vi "Create.vi"(8 "error in (no error)":errorcluster, 10 "GPIO":refnum<class "GPIO.lvclass">, 11 "ADC #":T1=-1) -> (0 "error out":errorcluster, 3 "AnalogIn out":refnum<class "AI.lvclass">)   [LabVIEW 2024, in "CTI.lvlib" / "AI.lvclass"]
uses:
  AI.lvclass
  ADC Number.ctl
  GPIO/GPIO.lvclass
  AI.lvclass/AI.ctl
  CTI.lvlib
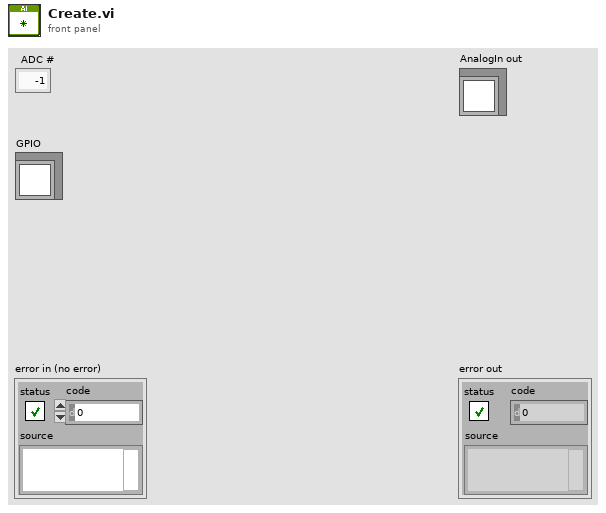
[diagram p1: front panel]
types:
  T1 = typedef "CTI.lvlib/ADC Number.ctl" = i8
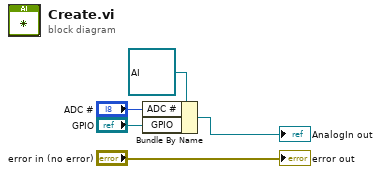
[diagram p0: block diagram]
diagram:
  n1 = Bundle By Name(cluster=refnum<class "AI.lvclass"> refnum ("AnalogIn in"), "ADC #"="ADC #", "GPIO"="GPIO") -> (→"AnalogIn out":refnum<class "AI.lvclass">)
  "error out" <- "error in (no error)"
